vi "Lidar Main V5.2 Unified.vi"() -> ()   [LabVIEW 2015]
uses:
  <vilib>/FPGAPlugInAG/PXIe-7962R/niLvFpga_Open_PXIe-7962R.vi
  <vilib>/rvi/interface/common/dynamic/niFpgaDynamicAddResources.vi
  <vilib>/FPGAPlugInAG/Dynamic/niLvFpga_Abort_Dynamic.vi
  <vilib>/rvi/interface/common/niFpgaWaitOnOcc.vi
  <vilib>/Utility/error.llb/Error Cluster From Error Code.vi
  <vilib>/FPGAPlugInAG/Dynamic/niLvFpga_Run_Dynamic.vi
  <vilib>/rvi/errors/niLvFpgaAdjustHostInterfaceError.vi
  <vilib>/FPGAPlugInAG/Dynamic/niLvFpga_Close_Dynamic.vi
  <vilib>/rvi/interface/nirviOpenFPGA/nirviOpenFPGA.xnode
  FPGA Bitfiles/Lidar Unified V5.2.1.lvbitx
  <vilib>/rvi/interface/nirviMethod/nirviMethod.xnode
  <vilib>/rvi/interface/nirviReadWriteControl/nirviReadWriteControl.xnode
  <vilib>/rvi/interface/nirviCloseFPGA/nirviCloseFPGA.xnode
  <vilib>/rvi/errors/niLvFpgaMergeErrorWithErrorCode.vi
  NiFpgaLv.dll
  <vilib>/rvi/interface/Simulation/niFpgaSimulationCallBeginRW.vi
  <vilib>/FPGAPlugInAG/Dynamic/niLvFpga_ReadFifo_Dynamic.vi
  <vilib>/FPGAPlugInAG/Dynamic/niLvFpga_ConfigureFifo_Dynamic.vi
  <vilib>/FPGAPlugInAG/Dynamic/niLvFpga_StartFifo_Dynamic.vi
panel:
  out "Version":string caption="Version:"
  in  "Laser Enable":bool=TRUE
  in  "VgaStart":u8
  out "data out":string
  in  "milliseconds to wait":u32=200
  in  "Frame Rate":u16=1247
  out "fps":u32
  out "PLL Locked 2":bool
  out "error out 3":errorcluster
  out "PLL Locked":bool
  in  "Matlab":bool=TRUE
  out "InitState":u8
  in  "local port":u16=2057
  in  "Matlab IP address":string="10.0.0.18"
  out "RawData":i32[](array[numeric])
  out "error out":errorcluster
  in  "Set VGA Const.":bool
  in  "VGA Val":i16
  out "String":string
  in  "Delay&Close":bool
  in  "SaveToFile":bool
  in  "StartAcq":u16=26 caption="Start Acq."
  in  "ActiveSensDeb":u8 caption="Active Sensor"
  in  "SensScanDeb":bool caption="Sensor Scan"
  in  "Active VCSL":u16
  in  "LedScanDebEn":bool=TRUE caption="VCSL Scan"
  in  "Fill VGA":bool
  in  "VGA data":i16[](array[numeric])=[15000, 15000, 15000, 15000, 15000, 15000, 15000, 15000, 15000, 15000, 15000, 15000, 15000, 15000, 15000, 15000, 15000, 15000, 15000, 15000, 15000, 15000, 15000, 15000, 15000, 15000, 15000, 15000, 15000, 15000, 15000, 15000, 15000, 15000, 15000, 15000, 15000, 15000, 15000, 15000, 15000, 15000, 15000, 15000, 15000, 15000, 15000, 15000, 15000, 15000, 15000, 15000, 15000, 15000, 15000, 15000, 15000, 15000, 15000, 15000, 15000, 15000, 15000, 15000, 15000, 15000, 15000, 15000, 15000, 15000, 15000, 15000, 15000, 15000, 15000, 15000, 15000, 15000, 15000, 15000, 15000, 15000, 15000, 15000, 15000, 15000, 15000, 15000, 15000, 15000, 15000, 15000, 15000, 15000, 15000, 15000, 15000, 15000, 15000, 15000]
  in  "PulseEnd":u16=25
  in  "StartPulse":u16=20
  in  "StartES":u16=38
  in  "StopES":u16=44
  in  "SamplingEnable":bool caption="Acquire Frames no Graph"
  in  "AcqMode":bool caption="Acq. Mode (T=Raw)"
  in  "SingleFrame":bool caption="Acquire Single Frame"
  out "Samples Amount":i32
  in  "Go":bool=TRUE caption="Acquire Frames With Graph"
  out "File Error":errorcluster
  in  "CloseFile":bool
  in  "OpenFile":bool
  out "Elements Remaining":u32
  out "Data":dbl[][](graph)
  in  "stop":bool
  out "FPGA Error":errorcluster
  # "Acquisition Control"
  # "Timing Control"
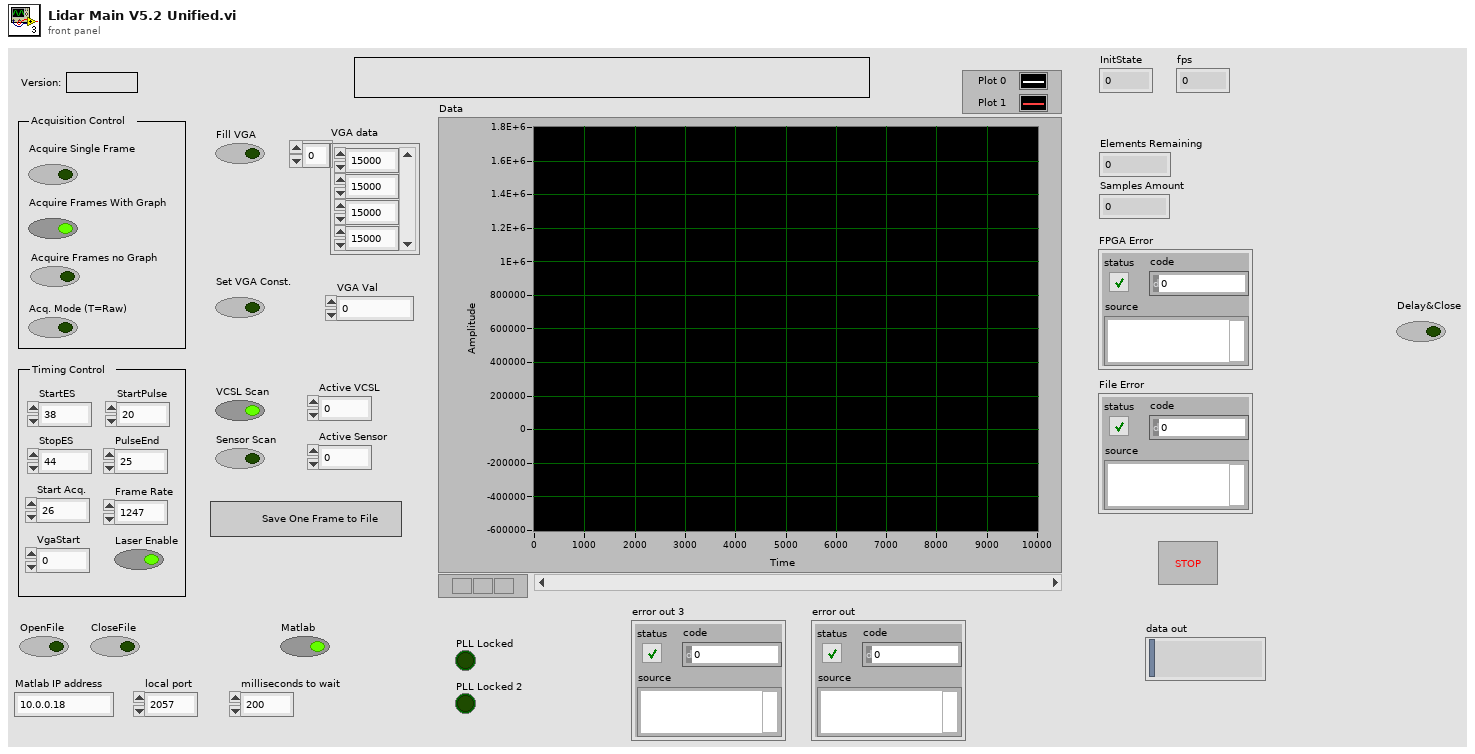
[diagram p1: front panel]
types:
  T1 = typedef "FpgaSlaveRef Unified Typedef.ctl" = refnum<k20>
  T2 = enum16{"open", "replace", "create", "open or create", "replace or create", "replace or create with confirmation"}
  T3 = enum16{"big-endian, network order", "native, host order", "little-endian"}
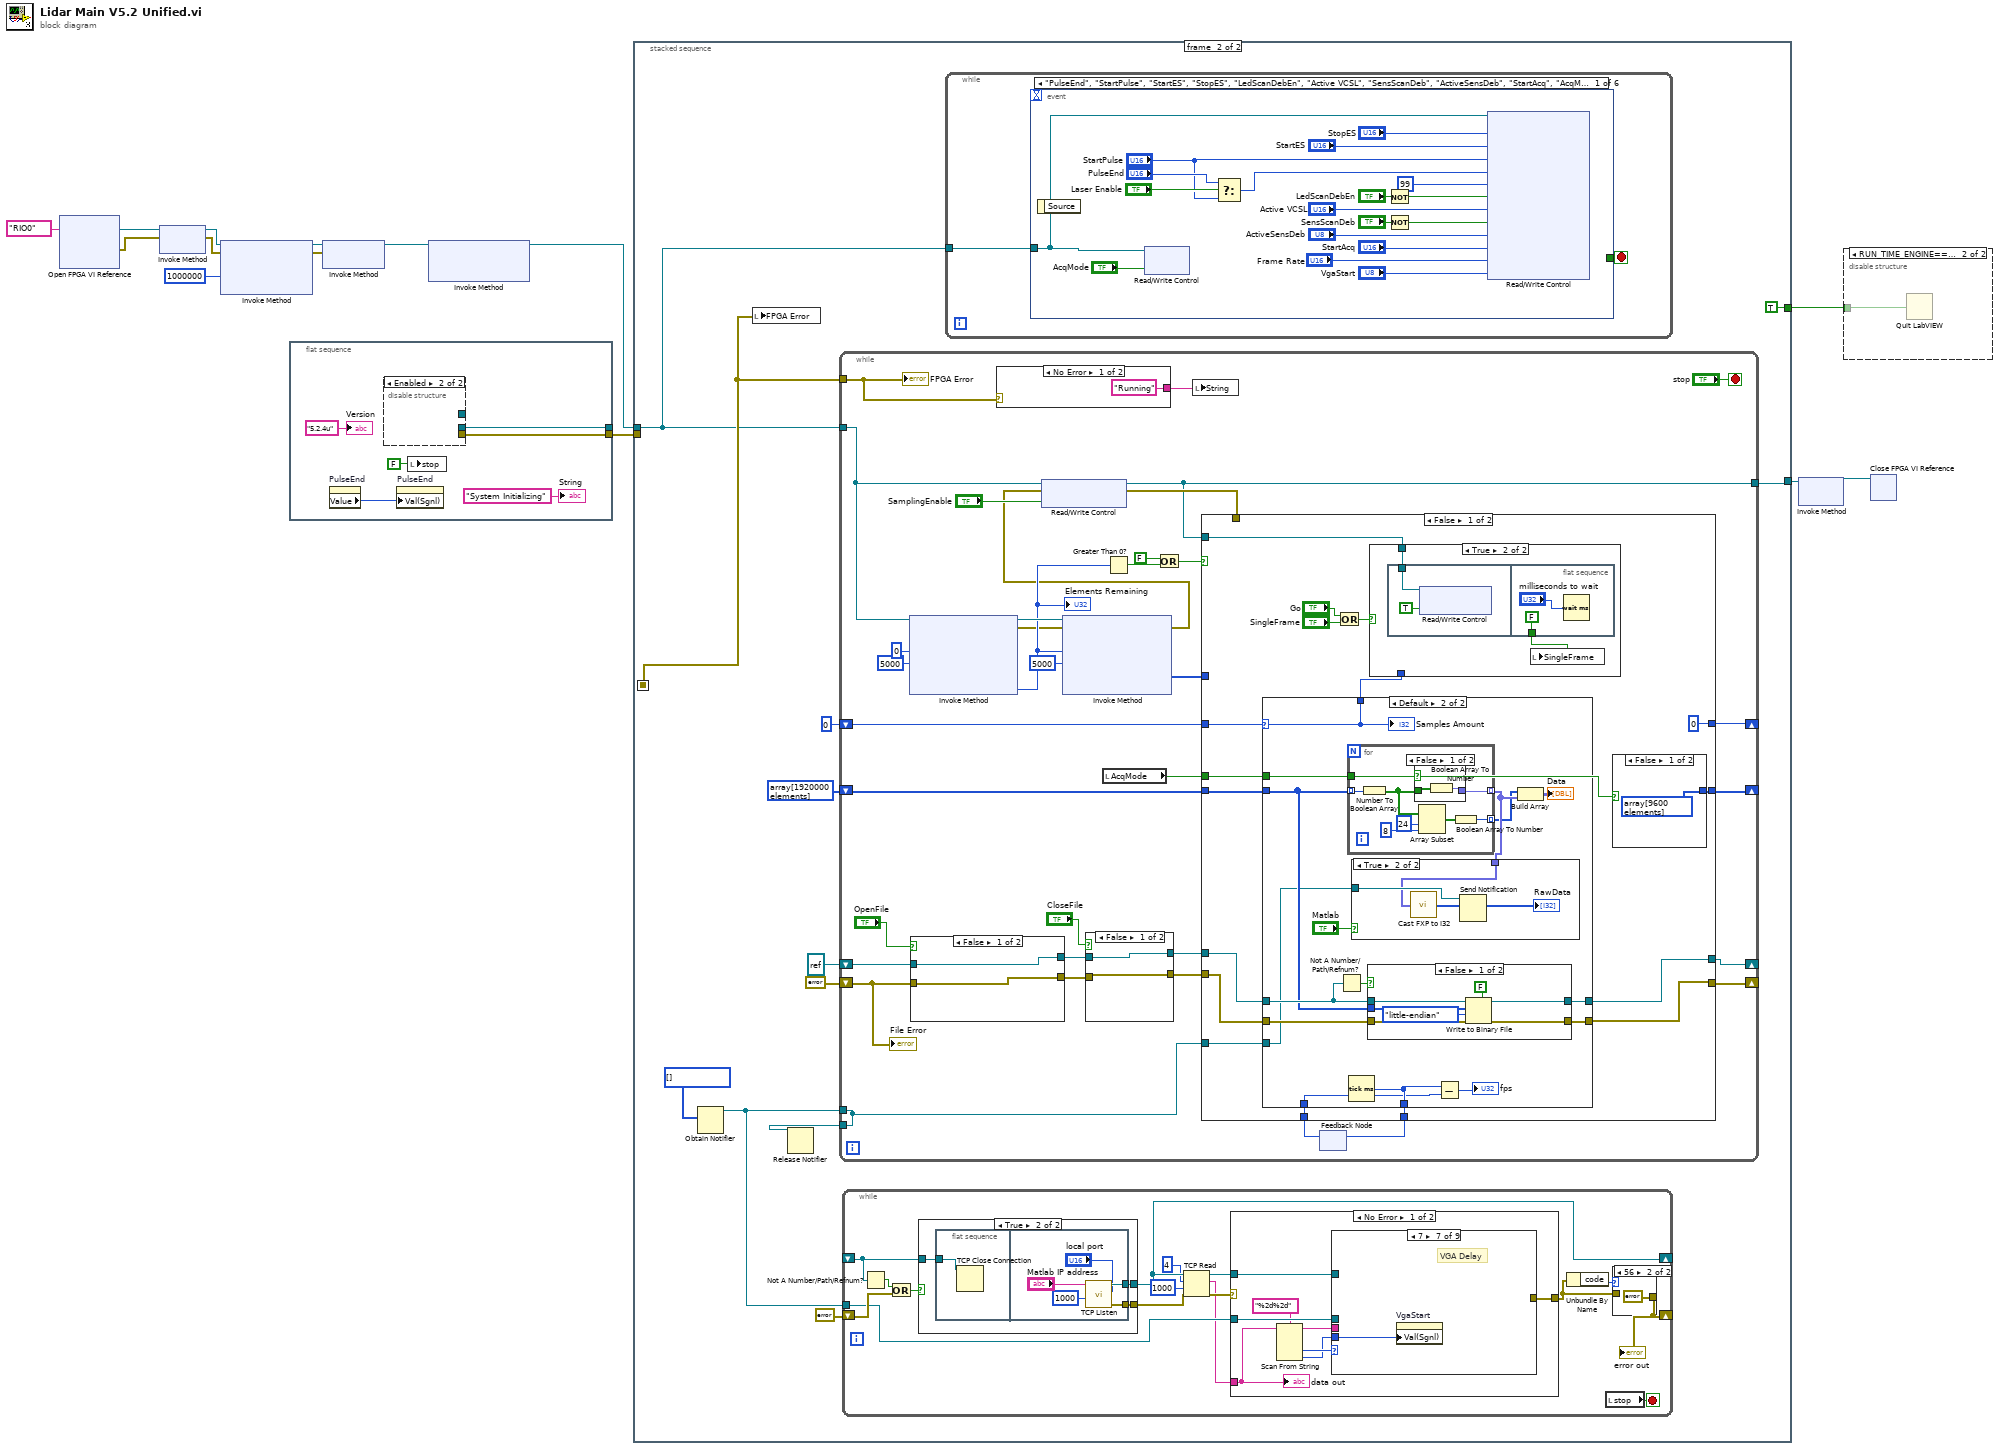
[diagram p0: block diagram]
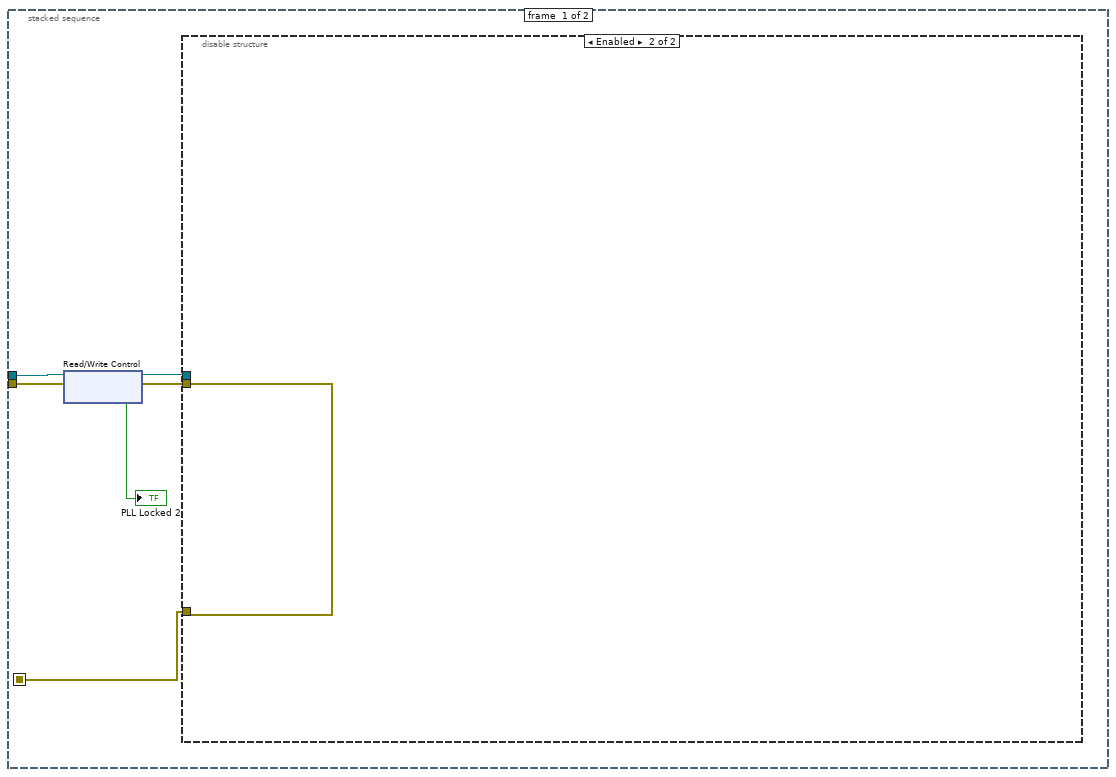
[diagram p3: hidden frame]
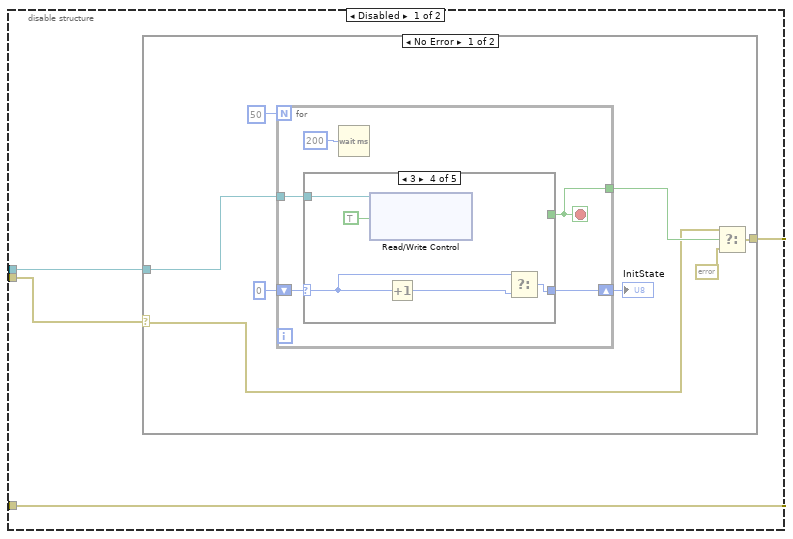
[diagram p4: hidden frame]
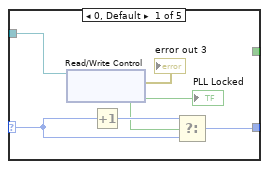
[diagram p5: hidden frame]
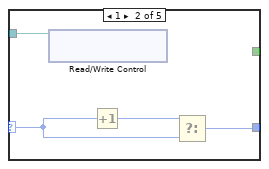
[diagram p6: hidden frame]
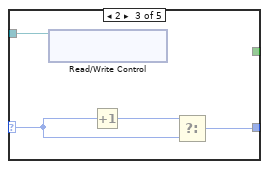
[diagram p7: hidden frame]
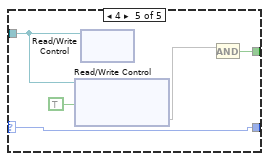
[diagram p8: hidden frame]
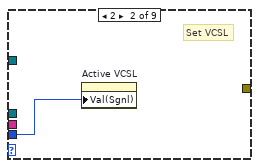
[diagram p13: hidden frame]
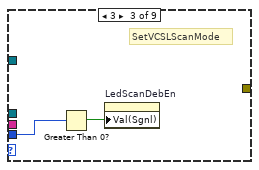
[diagram p14: hidden frame]
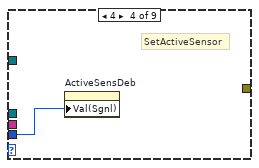
[diagram p15: hidden frame]
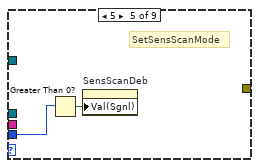
[diagram p16: hidden frame]
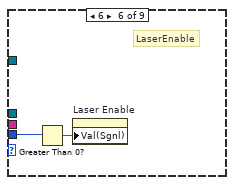
[diagram p17: hidden frame]
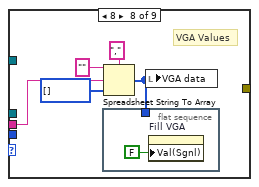
[diagram p18: hidden frame]
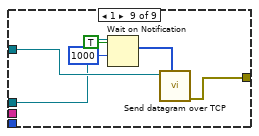
[diagram p19: hidden frame]
diagram:
  n1 = xnode "Open FPGA VI Reference"("resource name"=tag "RIO0") -> ("FPGA VI Reference Out"=w3:refnum<k20>, "error out"=w2:errorcluster)  [unwired: 1 in]
  n2 = xnode "Invoke Method"("FPGA VI Reference In"=w3, "error in"=w2) -> ("FPGA VI Reference Out"=w6:refnum<k20>, "error out"=w8:errorcluster)
  n3 = xnode "Invoke Method"("FPGA VI Reference In"=w6, "error in"=w8, "Requested Depth"=u32 1000000) -> ("FPGA VI Reference Out"=w9:refnum<k20>, "error out"=w10:errorcluster)  [unwired: 1 out]
  n4 = flat-sequence {
    tunnel: [w15] -> w14
    tunnel: [w16] -> _
    frame #0 {
      n5 = property on="PulseEnd" class="DigNum (strict)"() -> ("Value"=w19:u16)  [unwired: 2 in, 2 out]
      n6 = disable-structure shown="Enabled" {
        disable-tunnel: [w23 _] -> _
        disable-tunnel: [w22 _] -> w16
        disable-tunnel: [w21 _] -> w15
        frame Disabled {
          n7 = call "Open FPGA V5.2 Unified.vi"() -> ("error out"=w21:errorcluster, "SlaveRef"=w22:T1, "P2P ref"=w23:refnum<k20>)  [unwired: 8 in, 1 out]
        }
        frame Enabled {
        }
      }
      n8 = property on="PulseEnd" class="DigNum (strict)"("Val(Sgnl)"=w19) -> ()  [unwired: 2 in, 2 out]
      n9 = local write "stop"(FALSE ("stop")) -> ()
      "String" <- "System Initializing" ("String")
      "Version" <- "5.2.4u" ("Version")
    }
  }
  n10 = xnode "Invoke Method"("FPGA VI Reference In"=w9, "error in"=w10) -> ("FPGA VI Reference Out"=w5:refnum<k20>)  [unwired: 1 out]
  n11 = xnode "Invoke Method"("FPGA VI Reference In"=w5) -> ("FPGA VI Reference Out"=w4:refnum<k20>)  [unwired: 2 in, 1 out]
  n12 = stacked-sequence {
    seq-local: [w29 _] -> [_ w78]
    tunnel: w14 -> [w25 _]
    tunnel: w4 -> [w27 w77]
    tunnel: [_ w79] -> w13
    tunnel: [_ TRUE ("quit? (T)")] -> w12
    frame #0 {
      n13 = xnode "Read/Write Control"("FPGA VI Reference In"=w27, "error in"=w25) -> ("FPGA VI Reference Out"=w26:refnum<k20>, "error out"=w24:errorcluster, "PLL Locked"=→"PLL Locked 2":bool)
      n14 = disable-structure shown="Enabled" {
        disable-tunnel: w26 -> [w32 _]
        disable-tunnel: w24 -> [w31 w71]
        disable-tunnel: [w30 w71] -> w29
        frame Disabled {
          n15 = case shown="No Error" w31 {
            selector: w31 -> [w36 w70]
            tunnel: w32 -> [w40 _]
            tunnel: [w34 w70] -> w30
            frame No Error {
              n16 = for {
                N: 50 -> [_]
                shift-right: [w43] -> w33
                shift-left: u8 0 -> [w45]
                tunnel: w40 -> [w44]
                tunnel: [w41] -> w37
                stop <- w41 stop-if-true
                n17 = case shown="3" w45 {
                  selector: w45 -> [w50 w54 w58 w62 w66]
                  tunnel: w44 -> [w46 w52 w56 w63 w65]
                  tunnel: [w51 w55 w59 w64 w66] -> w43
                  tunnel: [_ _ _ _ w67] -> w41
                  frame 0, Default {
                    n18 = xnode "Read/Write Control"("FPGA VI Reference In"=w46) -> ("error out"=→"error out 3":errorcluster, "PLL Locked"=w48:bool)  [unwired: 1 in, 1 out]
                    "PLL Locked" <- w48
                    n19 = Increment(x=w50) -> (x+1=w49:u8)
                    n20 = Select(t=w49, s=w48, f=w50) -> (s? t:f=w51:u8)
                  }
                  frame 1 {
                    n21 = xnode "Read/Write Control"("FPGA VI Reference In"=w52) -> ()  [unwired: 1 in, 3 out]
                    n22 = Increment(x=w54) -> (x+1=w53:u8)
                    n23 = Select(t=w53, f=w54) -> (s? t:f=w55:u8)  [unwired: 1 in]
                  }
                  frame 2 {
                    n24 = xnode "Read/Write Control"("FPGA VI Reference In"=w56) -> ()  [unwired: 1 in, 3 out]
                    n25 = Increment(x=w58) -> (x+1=w57:u8)
                    n26 = Select(t=w57, f=w58) -> (s? t:f=w59:u8)  [unwired: 1 in]
                  }
                  frame 3 {
                    n27 = xnode "Read/Write Control"("FPGA VI Reference In"=w63, "StartSyncAction"=TRUE) -> ()  [unwired: 1 in, 3 out]
                    n28 = Increment(x=w62) -> (x+1=w61:u8)
                    n29 = Select(t=w62, f=w61) -> (s? t:f=w64:u8)  [unwired: 1 in]
                  }
                  frame 4 {
                    n30 = xnode "Read/Write Control"("FPGA VI Reference In"=w65, "StartSyncLoop"=TRUE ("StartSyncAction")) -> ("Trig1"=w68)  [unwired: 1 in, 2 out]
                    n31 = xnode "Read/Write Control"("FPGA VI Reference In"=w65) -> ()  [unwired: 1 in, 3 out]
                    n32 = And(x=w68) -> (x .and. y?=w67:bool)  [unwired: 1 in]
                  }
                }
                n33 = Wait (ms)(milliseconds to wait=u32 200) -> ()  [unwired: 1 out]
              }
              "InitState" <- w33
              n34 = Select(t=w36, s=w37, f=errorcluster {"status"=TRUE, "code"=0, "source"="Init Error"}) -> (s? t:f=w34:errorcluster)
            }
            frame Error {
            }
          }
        }
        frame Enabled {
        }
      }
    }
    frame #1 {
      n35 = Obtain Notifier(notification data type=u32[] []) -> (notifier out=w74:refnum<notifier>)  [unwired: 3 in, 2 out]
      n36 = local write "FPGA Error"(w78) -> ()
      n37 = while {
        tunnel: w78 -> [w199]
        tunnel: w77 -> [w192]
        shift-right: [w218] -> _
        shift-left: refnum<file> refnum ("refnum out") -> [w217]
        shift-right: [w215] -> _
        shift-left: errorcluster {"status"=FALSE, "code"=0, "source"=""} ("error out") -> [w214]
        shift-right: [w210] -> _
        shift-left: u32[] array[1920000 elements] -> [w212]
        shift-right: [w211] -> _
        shift-left: 0 -> [w207]
        tunnel: [w188] -> w79
        tunnel: w74 -> [w197]
        tunnel: [w197] -> w73
        stop <- "stop" stop-if-true
        n38 = xnode "Invoke Method"("FPGA VI Reference In"=w192, "Number of Elements"=u32 0, "Timeout (ms)"=5000) -> ("FPGA VI Reference Out"=w221:refnum<k20>, "error out"=w193:errorcluster, "Elements Remaining"=w206:u32)  [unwired: 1 in, 1 out]
        "Elements Remaining" <- w206
        n39 = case shown="False" "OpenFile" {
          tunnel: [w231 w236] -> w201
          tunnel: w217 -> [w231 _]
          tunnel: w214 -> [w230 _]
          tunnel: [w230 w235] -> w200
          frame False {
          }
          frame True {
            n40 = local write "OpenFile"(FALSE ("OpenFile")) -> ()
            n41 = Open/Create/Replace File(operation (0:open)=T2."open or create", disable buffering (F)=FALSE) -> (refnum out=w236:refnum<file>, error out=w235:errorcluster)  [unwired: 4 in, 1 out]
          }
        }
        n42 = case shown="No Error" w199 {
          tunnel: ["Running" ("String") "Error Initalizing" ("String")] -> w198
          frame No Error {
          }
          frame Error {
          }
        }
        n43 = xnode "Invoke Method"("FPGA VI Reference In"=w221, "error in"=w193, "Number of Elements"=w206, "Timeout (ms)"=5000) -> ("error out"=w190:errorcluster, "Data"=w219:u32[])  [unwired: 2 out]
        n44 = xnode "Read/Write Control"("FPGA VI Reference In"=w192, "error in"=w190, "Samplin|Enable"="SamplingEnable") -> ("FPGA VI Reference Out"=w188:refnum<k20>, "error out"=w189:errorcluster)
        n45 = case shown="False" "CloseFile" {
          tunnel: w201 -> [w226 w229]
          tunnel: [w226 _] -> w216
          tunnel: w200 -> [w225 w228]
          tunnel: [w225 _] -> w213
          frame False {
          }
          frame True {
            n46 = local write "CloseFile"(FALSE ("CloseFile")) -> ()
            n47 = Close File(refnum=w229, error in=w228) -> ()  [unwired: 2 out]
          }
        }
        n48 = local read "AcqMode"() -> (w196:bool)
        n49 = Greater Than 0?(x=w206) -> (x > 0?=w205:bool)
        n50 = Or(x=FALSE, y=w205) -> (x .or. y?=w204:bool)
        n51 = local write "String"(w198) -> ()
        n52 = feedback #1() -> (w194:u32)  [unwired: 1 in]
        n53 = case shown="False" w204 {
          tunnel: w219 -> [_ w306]
          tunnel: w216 -> [w247 w308]
          tunnel: [w246 w308] -> w218
          tunnel: [w244 w307] -> w215
          tunnel: w213 -> [w245 w307]
          tunnel: w212 -> [w250 w311]
          tunnel: w188 -> [w253 _]
          tunnel: [0 w312] -> w211
          tunnel: w207 -> [w251 w309]
          tunnel: [w249 w310] -> w210
          tunnel: w197 -> [w240 _]
          tunnel: w196 -> [w239 _]
          tunnel: [w238 w305] -> w195
          tunnel: w194 -> [w237 w305]
          tunnel: w189 -> [_ _]
          frame False {
            n54 = case shown="Default" w251 {
              selector: w251 -> [_ w269]
              tunnel: w250 -> [_ w268]
              tunnel: [_ w269] -> w248
              tunnel: w247 -> [w258 w270]
              tunnel: [w258 w274] -> w246
              tunnel: w245 -> [w257 w273]
              tunnel: [w257 w272] -> w244
              tunnel: w240 -> [_ w264]
              tunnel: w239 -> [_ w267]
              tunnel: [w256 w262] -> w238
              tunnel: w237 -> [w256 w261]
              frame 0 {
              }
              frame Default {
                n55 = Not A Number/Path/Refnum?(number/path/refnum=w270) -> (NaN/Path/Refnum?=w271:bool)
                n56 = for {
                  tunnel: w268 -> [w278] mode=indexing
                  tunnel: [w276] -> w260 mode=indexing
                  tunnel: [w277] -> w266 mode=indexing
                  tunnel: w267 -> [w275]
                  n57 = Number To Boolean Array(number=w278) -> (Boolean array=w279:bool[])
                  n58 = case shown="False" w275 {
                    tunnel: w279 -> [w284 w286]
                    tunnel: [w283 w285] -> w277
                    frame False {
                      n59 = Boolean Array To Number(Boolean array=w284) -> (number=w283:fxp<+/-,22,22>)
                    }
                    frame True {
                      n60 = Boolean Array To Number(Boolean array=w286) -> (number=w285:i16)
                    }
                  }
                  n61 = Array Subset(array=w279, index=24, length=8) -> (w280:bool[])
                  n62 = Boolean Array To Number(Boolean array=w280) -> (number=w276:u8)
                }
                n63 = Tick Count (ms)() -> (millisecond timer value=w262:u32)
                n64 = case shown="True" "Matlab" {
                  tunnel: w266 -> [_ w287]
                  tunnel: w264 -> [_ w289]
                  frame False {
                  }
                  frame True {
                    n65 = call "Cast FXP to I32.vi"("Array in"=w287) -> ("Array out"=w288:i32[])  [unwired: 4 in]
                    "RawData" <- w288
                    n66 = Send Notification(notification=w288, notifier=w289) -> ()  [unwired: 1 in, 2 out]
                  }
                }
                n67 = case shown="False" w271 {
                  tunnel: w270 -> [w296 w298]
                  tunnel: [w295 w298] -> w274
                  tunnel: w268 -> [w294 _]
                  tunnel: w273 -> [w293 w297]
                  tunnel: [w292 w297] -> w272
                  frame False {
                    n68 = Write to Binary File(file (use dialog)=w296, data=w294, error in=w293, 5:FALSE ("prepend array or string size? (T)"), 9:T3."little-endian" ("byte order (0:big-endian, network order)")) -> (refnum out=w295:refnum<file>, error out=w292:errorcluster)  [unwired: 1 in, 1 out]
                  }
                  frame True {
                  }
                }
                n69 = Subtract(x=w262, y=w261) -> (x-y=→"fps":u32)
                n70 = Build Array(w260, w266) -> (→"Data":fxp<+/-,22,22>[][])
                "Samples Amount" <- w269
              }
            }
            n71 = Or(x="Go", y="SingleFrame") -> (x .or. y?=w241:bool)
            n72 = case shown="True" w241 {
              tunnel: w253 -> [_ w300]
              tunnel: w248 -> [_ _]
              frame False {
              }
              frame True {
                n73 = flat-sequence {
                  tunnel: w300 -> [w302]
                  tunnel: [FALSE ("SingleFrame")] -> w299
                  frame #0 {
                    n74 = xnode "Read/Write Control"("FPGA VI Reference In"=w302, "SingleFrame"=TRUE) -> ()  [unwired: 1 in, 2 out]
                  }
                  frame #1 {
                    n75 = Wait (ms)(milliseconds to wait="milliseconds to wait") -> ()  [unwired: 1 out]
                  }
                }
                n76 = local write "SingleFrame"(w299) -> ()
              }
            }
            n77 = case shown="False" w239 {
              tunnel: [u32[] array[9600 elements] u32[] array[1920000 elements]] -> w249
              frame False {
              }
              frame True {
              }
            }
          }
          frame True {
            n78 = Array Size(array=w306) -> (size(s)=w313:i32)
            n79 = Add(x=w313, y=w309) -> (x+y=w312:i32)
            n80 = Replace Array Subset(array=w311, new element=w306, index=w309) -> (w310:u32[])
          }
        }
        n81 = feedback-in #1(w195) -> ()
        "File Error" <- w214
        "FPGA Error" <- w199
      }
      n82 = Release Notifier(notifier=w73) -> ()  [unwired: 2 in, 3 out]
      n83 = while {
        tunnel: w74 -> [w86]
        shift-right: [w96] -> _
        shift-left: _ -> [w95]
        shift-right: [w90] -> _
        shift-left: errorcluster {"status"=FALSE, "code"=0, "source"=""} ("error IO") -> [w93]
        stop <- w98 stop-if-true
        n84 = Not A Number/Path/Refnum?(number/path/refnum=w95) -> (NaN/Path/Refnum?=w94:bool)
        n85 = Or(x=w94, y=w93) -> (x .or. y?=w92:bool)
        n86 = case shown="True" w92 {
          tunnel: [w102 w105] -> w96
          tunnel: w95 -> [w102 w104]
          tunnel: [_ w103] -> w88
          frame False {
          }
          frame True {
            n87 = flat-sequence {
              tunnel: w104 -> [w106]
              tunnel: [w110] -> w105
              tunnel: [w107] -> w103
              frame #0 {
                n88 = TCP Close Connection(connection ID=w106) -> ()  [unwired: 2 in, 2 out]
              }
              frame #1 {
                n89 = call <vilib>:"TCP Listen.vi"("timeout ms (wait forever: -1)"=1000 ("timeout ms (60000)"), "port"="local port", "service name"="Matlab IP address") -> ("error out"=w107:errorcluster, "connection ID"=w110:refnum<k5>)  [unwired: 4 in, 3 out]
              }
            }
          }
        }
        n90 = TCP Read(connection ID=w96, bytes to read=4, error in (no error)=w88, 9:1000 ("timeout ms (25000)")) -> (connection ID out=w97:refnum<k5>, data out=w84:string, error out=w87:errorcluster)  [unwired: 1 in]
        n91 = case shown="No Error" w87 {
          selector: w87 -> [_ w141]
          tunnel: w97 -> [w119 _]
          tunnel: [w118 w141] -> w91
          tunnel: w86 -> [w117 _]
          tunnel: w84 -> [w116 _]
          frame No Error {
            n92 = Scan From String(format string="%2d%2d", input string=w116) -> (remaining string=w112:string, output 1=w114:i32, output 2=w113:i32)  [unwired: 4 in, 2 out]
            n93 = case shown="7" w114 {
              tunnel: w119 -> [_ _ _ _ _ _ _ _ w140]
              tunnel: [_ _ _ _ _ _ _ _ w139] -> w118
              tunnel: w117 -> [_ _ _ _ _ _ _ _ w138]
              tunnel: w113 -> [_ w120 w121 w123 w124 w127 w128 _ _]
              tunnel: w112 -> [_ _ _ _ _ _ _ w133 _]
              frame Default {
              }
              frame 2 {
                # "Set VCSL"
                n94 = property on="Active VCSL" class="DigNum (strict)"("Val(Sgnl)"=w120) -> ()  [unwired: 2 in, 2 out]
              }
              frame 3 {
                # "SetVCSLScanMode"
                n95 = Greater Than 0?(x=w121) -> (x > 0?=w122:bool)
                n96 = property on="LedScanDebEn" class="Bool (strict)"("Val(Sgnl)"=w122) -> ()  [unwired: 2 in, 2 out]
              }
              frame 4 {
                # "SetActiveSensor"
                n97 = property on="ActiveSensDeb" class="DigNum (strict)"("Val(Sgnl)"=w123) -> ()  [unwired: 2 in, 2 out]
              }
              frame 5 {
                # "SetSensScanMode"
                n98 = Greater Than 0?(x=w124) -> (x > 0?=w125:bool)
                n99 = property on="SensScanDeb" class="Bool (strict)"("Val(Sgnl)"=w125) -> ()  [unwired: 2 in, 2 out]
              }
              frame 6 {
                # "LaserEnable"
                n100 = Greater Than 0?(x=w127) -> (x > 0?=w126:bool)
                n101 = property on="Laser Enable" class="Bool (strict)"("Val(Sgnl)"=w126) -> ()  [unwired: 2 in, 2 out]
              }
              frame 7 {
                # "VGA Delay"
                n102 = property on="VgaStart" class="DigNum (strict)"("Val(Sgnl)"=w128) -> ()  [unwired: 2 in, 2 out]
              }
              frame 8 {
                # "VGA Values"
                n103 = flat-sequence {
                  tunnel: w129 -> [_]
                  frame #0 {
                    n104 = property on="Fill VGA" class="Bool (strict)"("Val(Sgnl)"=FALSE ("Value (Signaling)")) -> ()  [unwired: 2 in, 2 out]
                  }
                }
                n105 = Spreadsheet String To Array(delimiter (Tab)=",", format string="", spreadsheet string=w133, array type (2D Dbl)=i16[] []) -> (array=w129:i16[])
                n106 = local write "VGA data"(w129) -> ()
              }
              frame 1 {
                n107 = Wait on Notification(notifier=w138, ignore previous (F)=TRUE, timeout in ms (-1)=1000) -> (notification=w137:u32[])  [unwired: 1 in, 3 out]
                n108 = call "Send datagram over TCP.vi"("Data"=w137, "connection ID"=w140) -> ("error out"=w139:errorcluster)  [unwired: 9 in]
              }
            }
            "data out" <- w116
          }
          frame Error {
          }
        }
        n109 = Unbundle By Name(w91) -> ("code"=w85:i32)
        n110 = local read "stop"() -> (w98:bool)
        n111 = case shown="56" w85 {
          tunnel: w91 -> [w100 _]
          tunnel: [w100 errorcluster {"status"=FALSE, "code"=0, "source"=""} ("error IO")] -> w90
          frame Default {
          }
          frame 56 {
          }
        }
        "error out" <- w90
      }
      n112 = while {
        tunnel: w77 -> [w142]
        stop <- w143 stop-if-true
        n113 = event shown="[0] \"PulseEnd\", \"StartPulse\", \"StartES\", \"StopES\", \"LedScanDebEn\", \"Active VCSL\", \"SensScanDeb\", \"ActiveSensDeb\", \"StartAcq\", \"AcqMode\", \"Frame Rate\", \"VgaStart\", \"Laser Enable\": Value Change" {
          selector: _ -> [_ _ _ _ _ _]
          dyn-events: _ -> [_ _ _ _ _ _]
          timeout: _ -> [_ _ _ _ _ _]
          tunnel: [_ _ _ _ _ TRUE] -> w143
          tunnel: w142 -> [w156 _ _ _ w175 _]
          event "PulseEnd", "StartPulse", "StartES", "StopES", "LedScanDebEn", "Active VCSL", "SensScanDeb", "ActiveSensDeb", "StartAcq", "AcqMode", "Frame Rate", "VgaStart", "Laser Enable": Value Change {
            n114 = event-data() -> ()  [unwired: 1 in, 1 out]
            n115 = xnode "Read/Write Control"("FPGA VI Reference In"=w156, "Mode"="AcqMode") -> ()  [unwired: 1 in, 2 out]
            n116 = Select(t="PulseEnd", s="Laser Enable", f="StartPulse") -> (s? t:f=w147:u16)
            n117 = Not(x="LedScanDebEn") -> (.not. x?=w149:bool)
            n118 = Not(x="SensScanDeb") -> (.not. x?=w151:bool)
            n119 = xnode "Read/Write Control"("FPGA VI Reference In"=w156, "StopES"="StopES", "StartES"="StartES", "StartPulse"="StartPulse", "PulseEnd"=w147, "AiNoOfSamples"=u16 99, "LedScanDebEn"=w149, "ActiveLedIndexDeb"="Active VCSL", "SensScanDeb"=w151, "ActiveSensDeb"="ActiveSensDeb", "StartAcq"="StartAcq", "NoOfSamples"="Frame Rate", "StartVGA"="VgaStart") -> ()  [unwired: 1 in, 2 out]
          }
          event "Set VGA Const.": Value Change {
            n120 = event-data() -> ()  [unwired: 1 in, 6 out]
            n121 = for {
              N: 99 -> [_]
              tunnel: [w165] -> w162 mode=indexing
              tunnel: "VGA Val" -> [w165]
            }
            n122 = local write "VGA data"(w162) -> ()
          }
          event "SaveToFile": Value Change {
            n123 = event-data() -> ()  [unwired: 1 in, 1 out]
            n124 = flat-sequence {
              tunnel: [TRUE ("Value (Signaling)")] -> w170
              frame #0 {
                n125 = local write "Go"(FALSE ("Go")) -> ()
              }
            }
            n126 = property on="OpenFile" class="Bool (strict)"("Val(Sgnl)"=w170) -> (error out=w169:errorcluster)  [unwired: 2 in, 1 out]
            n127 = property on="SingleFrame" class="Bool (strict)"(error in=w169, "Val(Sgnl)"=TRUE ("Value (Signaling)")) -> (error out=w167:errorcluster)  [unwired: 1 in, 1 out]
            n128 = property on="Delay&Close" class="Bool (strict)"(error in=w167, "Val(Sgnl)"=FALSE ("Value (Signaling)")) -> ()  [unwired: 1 in, 2 out]
          }
          event "Delay&Close": Value Change {
            n129 = event-data() -> ()  [unwired: 1 in, 6 out]
            n130 = flat-sequence {
              frame #0 {
                n131 = Wait (ms)(milliseconds to wait=u32 3000) -> ()  [unwired: 1 out]
              }
              frame #1 {
                n132 = local write "CloseFile"(TRUE ("CloseFile")) -> ()
              }
            }
          }
          event "Fill VGA": Value Change {
            n133 = event-data() -> ()  [unwired: 1 in, 1 out]
            n134 = for {
              tunnel: w175 -> [w183]
              tunnel: "VGA data" -> [w182] mode=indexing
              tunnel: [FALSE] -> w176
              i -> [w181]
              n135 = xnode "Read/Write Control"("FPGA VI Reference In"=w183, "VgaAdd"=w181, "VgaData"=w182, "FillVga"=TRUE) -> ("FPGA VI Reference Out"=w180:refnum<k20>)  [unwired: 1 in, 1 out]
              n136 = while {
                tunnel: w180 -> [w185]
                stop <- w184 continue-if-true
                n137 = xnode "Read/Write Control"("FPGA VI Reference In"=w185) -> ("FillVga"=w184:bool)  [unwired: 1 in, 2 out]
              }
            }
            n138 = local write "Fill VGA"(w176) -> ()
          }
          event "stop": Value Change {
            n139 = event-data() -> ()  [unwired: 1 in, 6 out]
          }
        }
      }
    }
  }
  n140 = xnode "Invoke Method"("FPGA VI Reference In"=w13) -> ("FPGA VI Reference Out"=w11:refnum<k20>)  [unwired: 1 in, 1 out]
  n141 = disable-structure shown="RUN_TIME_ENGINE==True" {
    disable-tunnel: w12 -> [_ w314]
    frame condition #0 (active) {
    }
    frame condition #1 {
      n142 = Quit LabVIEW(quit? (T)=w314) -> ()
    }
  }
  n143 = xnode "Close FPGA VI Reference"("FPGA VI Reference In"=w11) -> ()  [unwired: 1 in, 1 out]
